vi "SerialTest.vi"() -> ()   [LabVIEW 2017]
uses:
  <vilib>/MakerHub/LINX/Public/Peripherals/UART/UART Write String.vi
  <vilib>/MakerHub/LINX/Public/Peripherals/UART/UART Write Byte Array.vi
  <vilib>/MakerHub/LINX/Private/Local IO/LinxUartWrite.vi
  <vilib>/MakerHub/LINX/Public/Utilities/Check Channel.vi
  <vilib>/MakerHub/LINX/Public/Utilities/Open Serial.vi
  <vilib>/MakerHub/LINX/Private/Utilties/Generate Error.vi
  <vilib>/MakerHub/LINX/Public/Peripherals/UART/UART Read String.vi
  <vilib>/MakerHub/LINX/LMH-LINX.lvlib
panel:
  out "Data 2":string
  in  "Data":string
  in  "stop":bool
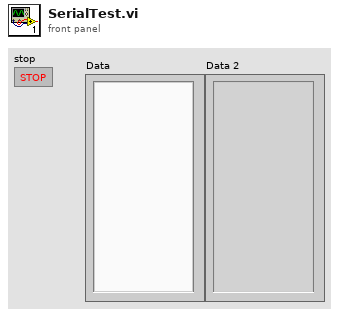
[diagram p1: front panel]
types:
  T1 = typedef "LMH-LINX.lvlib/LINX Ref.ctl" = cluster{"IO":T2, "Interface":T3, "LINX Device Config":T4}
  T2 = typedef "LMH-LINX.lvlib/Platform.ctl" = enum16{"Remote", "Local"}
  T3 = typedef "LMH-LINX.lvlib/Interface.ctl" = enum16{"Serial", "TCP"}
  T4 = typedef "LMH-LINX.lvlib/Device.lvlib/LINX Device Config.ctl" = cluster{"Interface":T3, "COM Port":refnum<visa-resource-name>, "TCP Configuration":T5, "Device Family":u8, "Device ID":u8, "Device Name":string, "TCP Ref":refnum<k5>, "Channels":T6}
  T5 = typedef "LMH-LINX.lvlib/Device.lvlib/TCP Config.ctl" = cluster{"IP Address":string, "Port":u16}
  T6 = typedef "LMH-LINX.lvlib/Channels.ctl" = cluster{"DI":u8[], "DO":u8[], "AI":u8[], "AO":u8[], "PWM":u8[], "QE":u8[], "UART":u8[], "I2C 2":u8[], "SPI":u8[], "CAN":u8[], "Servo":u8[], "AI Ref (V)":dbl, "AI Resolution (Bits)":u8, "AO Ref (V)":dbl, "AO Resolution (Bits)":u8}
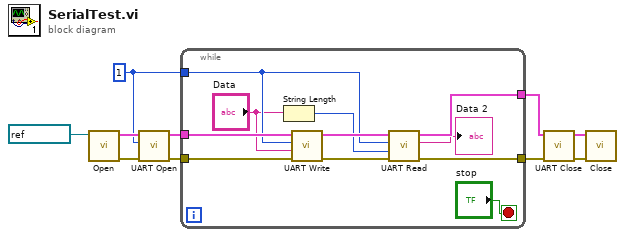
[diagram p0: block diagram]
diagram:
  w1 = u8 1 ("UART Channel (0)")
  n1 = call-poly <vilib>:"Open.vi"("Serial Port"=refnum<visa-resource-name> "COM3") -> ("Error Out"=w7:errorcluster, "LINX Resource"=w8:T1)  [unwired: 8 in, 1 out]
  n2 = call <vilib>:"UART Open.vi"("Error In"=w7, "UART Channel (0)"=w1, "LINX Resource"=w8) -> ("Error Out"=w3:errorcluster, "LINX Resource"=w5:T1)  [unwired: 6 in, 1 out]
  n3 = while {
    tunnel: w5 -> [w20]
    tunnel: [w18] -> w4
    tunnel: w3 -> [w17]
    tunnel: [w15] -> w2
    tunnel: w1 -> [w14]
    stop <- "stop" stop-if-true
    n4 = String Length(string="Data") -> (length=w13:i32)
    n5 = call-poly <vilib>:"UART Write.vi"("Error In"=w17, "Data"="Data", "UART Channel (0)"=w14, "LINX Resource"=w20) -> ("Error Out"=w16:errorcluster, "LINX Resource"=w19:T1)  [unwired: 6 in]
    n6 = call-poly <vilib>:"UART Read.vi"("Error In"=w16, "Num Bytes"=w13, "UART Channel (0)"=w14, "LINX Resource"=w19) -> ("Error Out"=w15:errorcluster, "Data"=→"Data 2":string, "LINX Resource"=w18:T1)  [unwired: 5 in]
  }
  n7 = call <vilib>:"UART Close.vi"("Error In"=w2, "LINX Resource"=w4) -> ("Error Out"=w9:errorcluster, "LINX Resource"=w10:T1)  [unwired: 8 in]
  n8 = call <vilib>:"Close.vi"("Error In"=w9, "LINX Resource"=w10) -> ()  [unwired: 9 in, 1 out]
